vi "Serve Buffers.vi"(8 "error in":errorcluster, 11 "data server thread in":refnum<class "Data Server Thread.lvclass">) -> (0 "error out":errorcluster, 3 "data server thread out":refnum<class "Data Server Thread.lvclass">)   [LabVIEW 2019, in "DSF Core.lvlib" / "Data Server Thread.lvclass"]
uses:
  Data Server Thread.lvclass
  Data Server Thread.lvclass/Data Server Thread.ctl
  <vilib>/NI/Memory Manager/Classes/Pointer/Pointer.lvclass/Pointer.ctl
  <vilib>/NI/Memory Manager/Classes/Pointer/Is Null.vi
  <vilib>/NI/Memory Manager/Classes/Pointer/Get Address.vi
  Status/Status Pointer.lvclass
  C:/Program Files (x86)/National Instruments/LabVIEW 2019/vi.lib/NI/Memory Manager/Classes/Pointer/Pointer.lvclass
  Buffer/Buffer.lvclass
  Buffer/Get Buffer Size.vi
  Buffer/Read Buffer 1D U8.vi
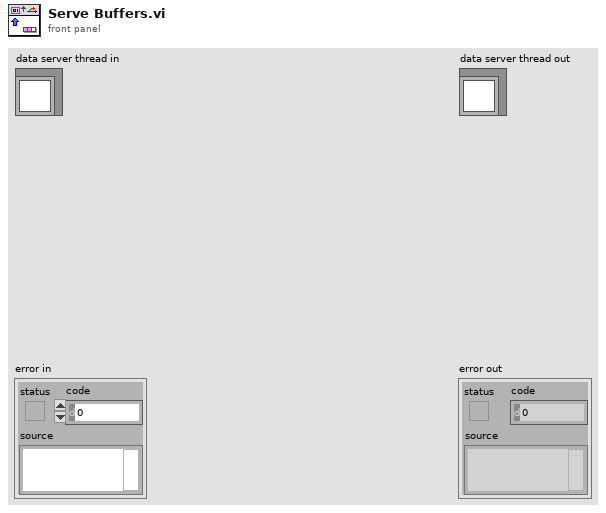
[diagram p1: front panel]
types:
  T1 = typedef "DSF Core.lvlib/Data Server Thread.lvclass/Viewer Data.ctl" = cluster{"remote address":string, "remote port":u16, "connection ID":refnum<k5>, "Buffer":refnum<class "Buffer.lvclass">, "Status":refnum<class "Status Pointer.lvclass">}
  T2 = typedef "DSF Core.lvlib/Status Pointer.lvclass/Status Data.ctl" = cluster{"duration":u64, "period":u64, "iteration":u64, "late count":u64}
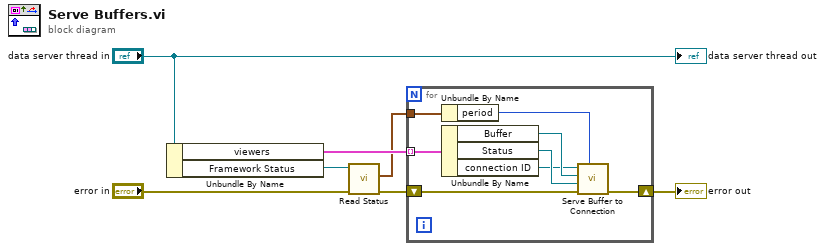
[diagram p0: block diagram]
diagram:
  n1 = Unbundle By Name("data server thread in") -> ("viewers"=w2:T1[], "Framework Status"=w3:refnum<class "Status Pointer.lvclass">)
  n2 = call "Read Status.vi"("error in (no error)"="error in", "status pointer in"=w3) -> ("error out"=w4:errorcluster, "status"=w1:T2)  [unwired: 7 in, 1 out]
  n3 = for {
    tunnel: w2 -> [w14] mode=indexing
    shift-right: [w15] -> w7
    shift-left: w4 -> [w13]
    tunnel: w1 -> [w9]
    n4 = Unbundle By Name(w9) -> ("period"=w8:u64)
    n5 = Unbundle By Name(w14) -> ("Buffer"=w12:refnum<class "Buffer.lvclass">, "Status"=w11:refnum<class "Status Pointer.lvclass">, "connection ID"=w10:refnum<k5>)
    n6 = call "Serve Buffer to Connection.vi"("framework period"=w8, "error in"=w13, "status"=w11, "buffer"=w12, "connection ID in"=w10) -> ("error out"=w15:errorcluster)  [unwired: 5 in, 1 out]
  }
  "error out" <- w7
  "data server thread out" <- "data server thread in"
